vi "write timeout.vi"(8 "error in (no error)":errorcluster, 10 "timeout ms":i32, 11 "Redis TCP Client in":refnum<class "Redis TCP Client.lvclass">) -> (0 "error out":errorcluster, 3 "Redis TCP Client out":refnum<class "Redis TCP Client.lvclass">)   [LabVIEW 2019, in "Redis Client for LabVIEW.lvlib" / "Redis TCP Client.lvclass"]
uses:
  Redis TCP Client.lvclass
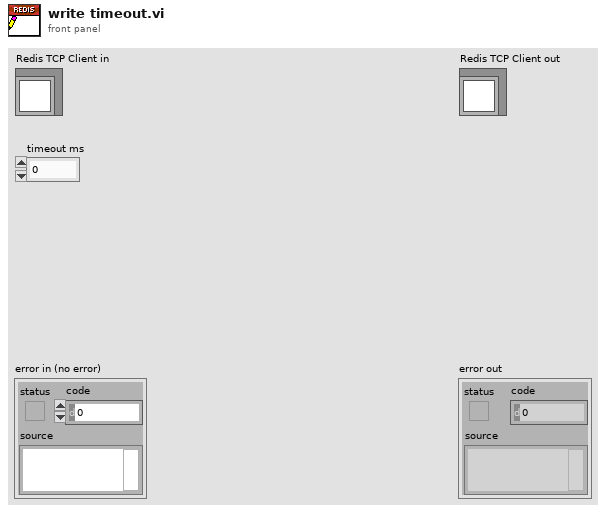
[diagram p1: front panel]
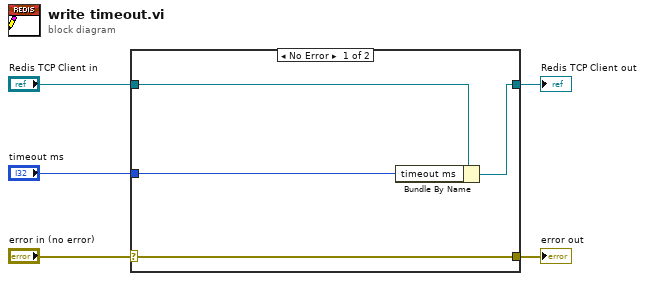
[diagram p0: block diagram]
diagram:
  n1 = case shown="No Error" "error in (no error)" {
    selector: "error in (no error)" -> [w9 w10]
    tunnel: [w9 w10] -> w4
    tunnel: [w7 w11] -> w2
    tunnel: "Redis TCP Client in" -> [w8 w11]
    tunnel: "timeout ms" -> [w6 _]
    frame No Error {
      n2 = Bundle By Name(cluster=w8, "timeout ms"=w6) -> (w7:refnum<class "Redis TCP Client.lvclass">)
    }
    frame Error {
    }
  }
  "error out" <- w4
  "Redis TCP Client out" <- w2
